vi "KickSkillVSS.vi"(8 "error in (no error)":errorcluster, 9 "BallRef":refnum<class "Ball.lvclass">, 10 "Robot":refnum<class "Robot.lvclass">, 11 "KickSkillVSS in":refnum<class "KickSkillVSS.lvclass">) -> (0 "error out":errorcluster, 2 "Robot out":refnum<class "Robot.lvclass">, 3 "KickSkillVSS out":refnum<class "KickSkillVSS.lvclass">)   [LabVIEW 2023, in "KickSkillVSS.lvclass"]
uses:
  KickSkillVSS.lvclass
  Robot_class/Robot.lvclass
  C:/Users/roboi/Downloads/VSS_AI-Larc2023/Object_class/Object.lvclass
  Ball_class/Ball.lvclass
  Field_class/Field.lvclass
  Utilities_class/Utilities.lvclass
  Object_class/Object.lvclass/Object.ctl
  Ball_class/Ball.lvclass/Ball.ctl
  Robot_class/Robot.lvclass/Robot.ctl
  Game_class/Navigation/VSSNavigation/VSSAttackerStates.ctl
  Object_class/Read x.vi
  Object_class/Read y.vi
  Ball_class/Read v_x.vi
  Ball_class/Read v_y.vi
  Object_class/Read pos_est_x.vi
  Object_class/Read pos_est_y.vi
  Robot_class/Read orientation.vi
  Robot_class/Write dest_x.vi
  Robot_class/Write dest_y.vi
  Robot_class/Write id.vi
panel:
  in  "Field":refnum<class "Field.lvclass">
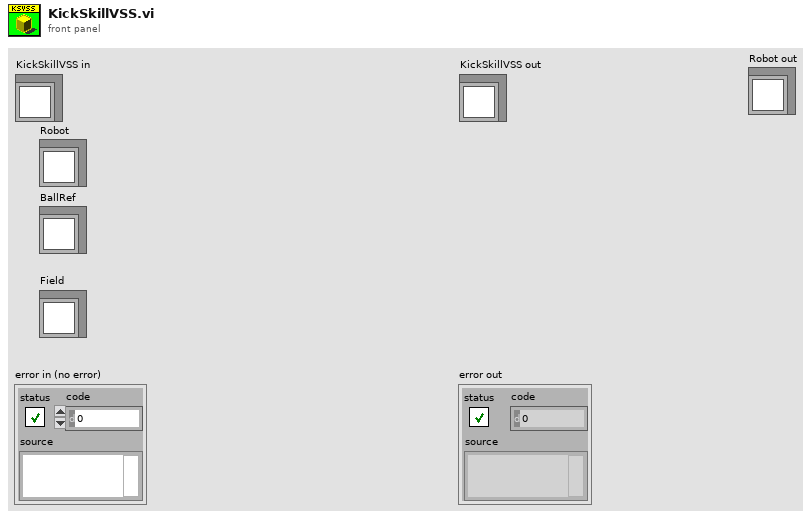
[diagram p1: front panel]
types:
  T1 = typedef "VSSAttackerStates.ctl" = enum16{"Pass", "GoToTangent", "BallGetting", "GoToKick", "Rotate anti-clockwise", "Rotate Clockwise", ""}
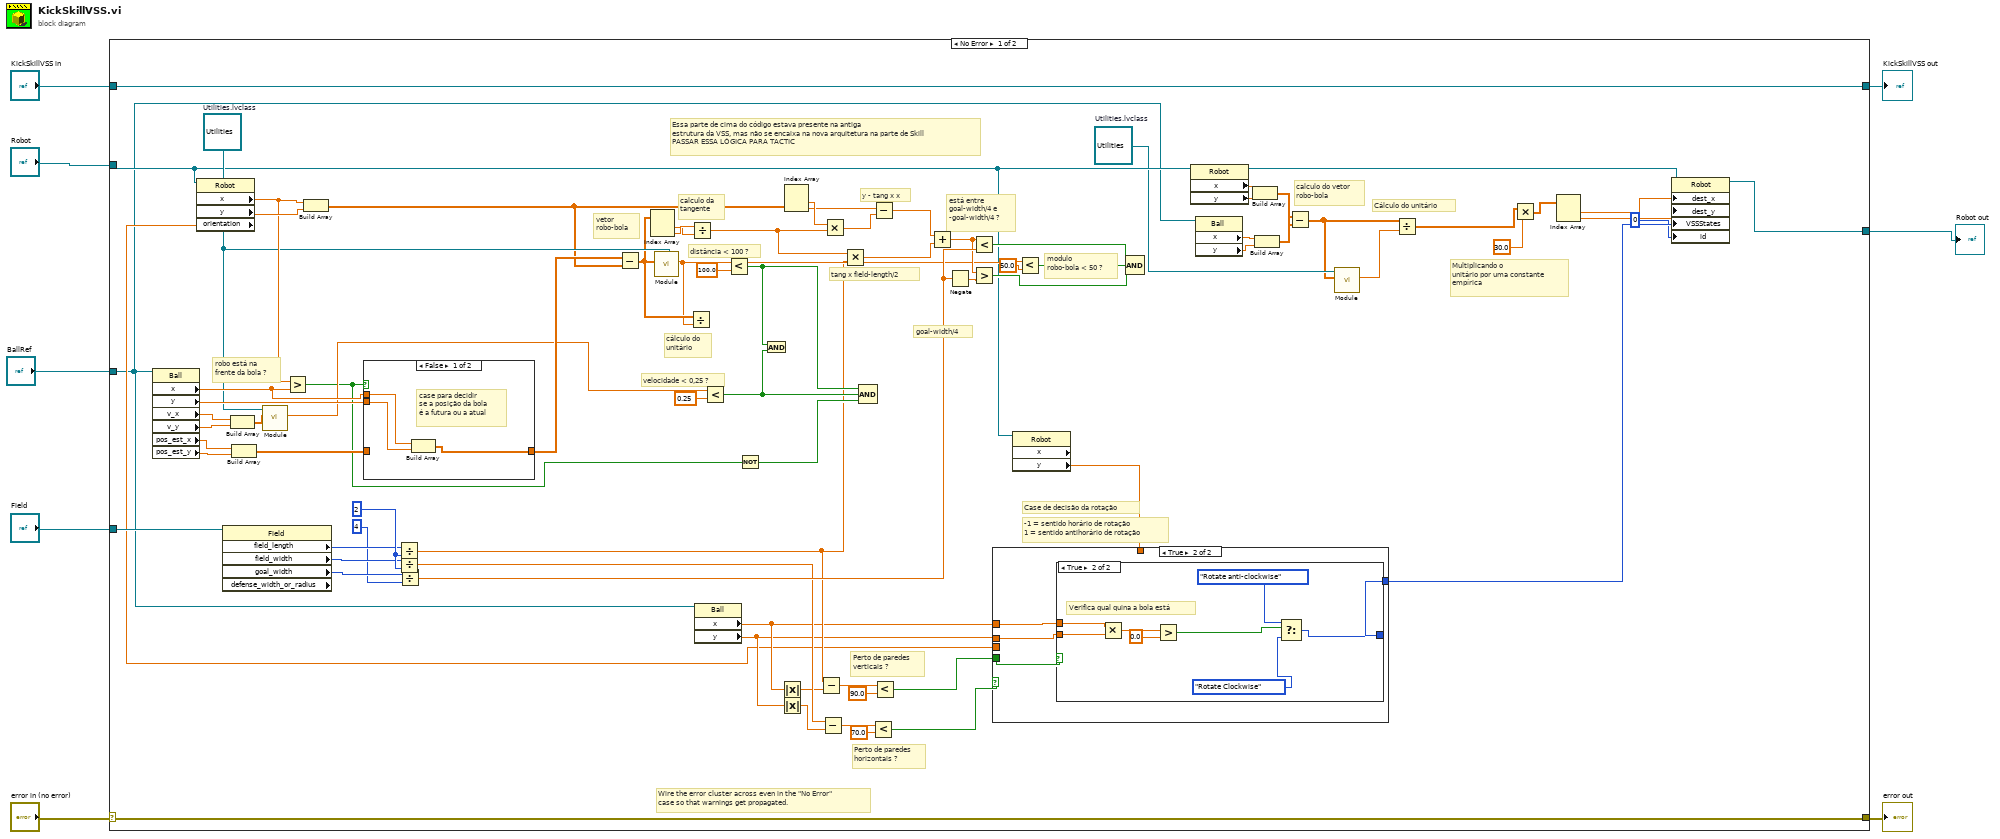
[diagram p0: block diagram]
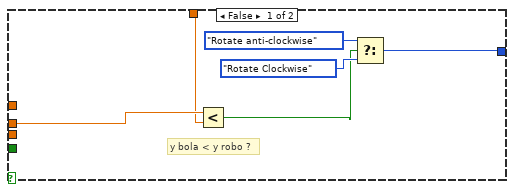
[diagram p2: hidden frame]
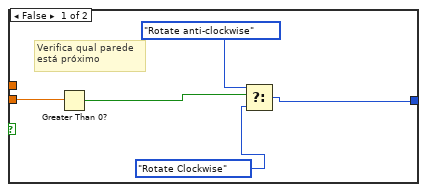
[diagram p3: hidden frame]
diagram:
  n1 = case shown="No Error" "error in (no error)" {
    selector: "error in (no error)" -> [w86 w117]
    tunnel: [w86 w117] -> w7
    tunnel: [w87 w116] -> w5
    tunnel: "KickSkillVSS in" -> [w87 w116]
    tunnel: "Robot" -> [w27 w115]
    tunnel: [w85 w115] -> w3
    tunnel: "BallRef" -> [w23 _]
    tunnel: "Field" -> [w66 _]
    frame No Error {
      w18 = refnum<class "Utilities.lvclass"> refnum  # Utilities.lvclass
      w59 = 2
      w73 = refnum<class "Utilities.lvclass"> refnum  # Utilities.lvclass
      # "Multiplicando o\nunitário por uma constante\nempírica"
      # "Cálculo do unitário"
      # "calculo do vetor\nrobo-bola"
      # "Essa parte de cima do código estava presente na antiga \nestrutura da VSS, mas não se encaixa na nova arquitetura na parte de Skill\nPASSAR ESSA LÓGICA PARA TACTIC"
      # "-1 = sentido horário de rotação\n1 = sentido antihorário de rotação"
      # "Case de decisão da rotação"
      # "Perto de paredes\nhorizontais ?"
      # "Perto de paredes\nverticais ?"
      # "modulo\nrobo-bola < 50 ?"
      # "está entre\ngoal-width/4 e\n-goal-width/4 ?"
      # "goal-width/4"
      # "y - tang x x"
      # "tang x field-length/2"
      # "velocidade < 0,25 ?"
      # "distância < 100 ?"
      # "cálculo do\nunitário"
      # "calculo da\ntangente"
      # "vetor \nrobo-bola"
      # "robo está na\nfrente da bola ?"
      # "Wire the error cluster across even in the \"No Error\"\ncase so that warnings get propagated."
      n2 = property class="Ball"(reference=w23) -> ("x"=w74:dbl, "y"=w75:dbl, "v_x"=w84:dbl, "v_y"=w83:dbl, "pos_est_x"=w81:dbl, "pos_est_y"=w80:dbl)  [unwired: 1 in, 2 out]
      n3 = property class="Robot"(reference=w27) -> ("x"=w78:dbl, "y"=w79:dbl, "orientation"=w28:dbl)  [unwired: 1 in, 2 out]
      n4 = property class="Field" props=["field_length", "field_width", "goal_width", "defense_width_or_radius"](reference=w66) -> ("field_length"=w58:i32, "field_width"=w57:i32, "goal_width"=w51:i32)  [unwired: 1 in, 3 out]
      n5 = Build Array(w84, w83) -> (w82:dbl[])
      n6 = Build Array(w81, w80) -> (w76:dbl[])
      n7 = call-dynamic "Module.vi"("2D vector"=w82, "Utilities in"=w73) -> ("Modulo"=w67:dbl)  [unwired: 7 in, 2 out]
      n8 = Greater?(x=w78, y=w74) -> (0:w64:bool)
      n9 = Build Array(w78, w79) -> (w65:dbl[])
      n10 = case shown="False" w64 {
        tunnel: [w111 w114] -> w77
        tunnel: w76 -> [_ w114]
        tunnel: w75 -> [w113 _]
        tunnel: w74 -> [w112 _]
        frame False {
          # "case para decidir \nse a posição da bola \né a futura ou a atual"
          n11 = Build Array(w112, w113) -> (w111:dbl[])
        }
        frame True {
        }
      }
      n12 = Divide(x=w58, y=w59) -> (x/y=w39:dbl)
      n13 = Divide(x=w57, y=w59) -> (x/y=w41:dbl)
      n14 = Divide(x=w51, y=4) -> (x/y=w49:dbl)
      n15 = Subtract(x=w77, y=w65) -> (x-y=w70:dbl[])
      n16 = Index Array(array=w70) -> (element #1=w71:dbl, element #2=w72:dbl)  [unwired: 2 in]
      n17 = call-dynamic "Module.vi"("2D vector"=w70, "Utilities in"=w73) -> ("Modulo"=w45:dbl)  [unwired: 7 in, 2 out]
      n18 = Divide(x=w70, y=w45) -> ()  [unwired: 1 out]
      n19 = Divide(x=w72, y=w71) -> (x/y=w60:dbl)
      n20 = property class="Ball"(reference=w23) -> ("x"=w31:dbl, "y"=w30:dbl)  [unwired: 1 in, 2 out]
      n21 = Less?(x=w67, y=0.25) -> (x < y?=w62:bool)
      n22 = Less?(x=w45, y=100.0) -> (x < y?=w63:bool)
      n23 = Not(x=w64) -> (.not. x?=w61:bool)
      n24 = And(x=w63, y=w62) -> ()  [unwired: 1 out]
      n25 = Absolute Value(x=w31) -> (abs(x)=w38:dbl)
      n26 = Absolute Value(x=w30) -> (abs(x)=w40:dbl)
      n27 = Index Array(array=w65) -> (element #1=w56:dbl, element #2=w55:dbl)  [unwired: 2 in]
      n28 = Subtract(x=w39, y=w38) -> (x-y=w37:dbl)
      n29 = Subtract(x=w41, y=w40) -> (x-y=w36:dbl)
      n30 = Multiply(x=w56, y=w60) -> (x*y=w54:dbl)
      n31 = Multiply(x=w60, y=w39) -> (x*y=w52:dbl)
      n32 = Compound Arithmetic op=AND(w63, w62, w61) -> ()  [unwired: 1 out]
      n33 = Less?(x=w36, y=70.0) -> (x < y?=w33:bool)
      n34 = Subtract(x=w55, y=w54) -> (x-y=w53:dbl)
      n35 = Less?(x=w37, y=90.0) -> (x < y?=w32:bool)
      n36 = Add(x=w53, y=w52) -> (x+y=w47:dbl)
      n37 = Negate(x=w49) -> (-x=w48:dbl)
      n38 = Less?(x=w47, y=w49) -> (x < y?=w43:bool)
      n39 = Greater?(x=w47, y=w48) -> (0:w42:bool)
      n40 = property class="Robot" props=["x", "y"](reference=w27) -> ("y"=w29:dbl)  [unwired: 1 in, 3 out]
      n41 = case shown="True" w33 {
        tunnel: w32 -> [_ w97]
        tunnel: w31 -> [_ w96]
        tunnel: w30 -> [w93 w95]
        tunnel: [w92 w94] -> w10
        tunnel: w29 -> [w91 _]
        tunnel: w28 -> [_ _]
        frame False {
          # "y bola < y robo ?"
          n42 = Less?(x=w93, y=w91) -> (x < y?=w88:bool)
          n43 = Select(t=VSSAttackerStates."Rotate anti-clockwise" ("VSSStates"), s=w88, f=VSSAttackerStates."Rotate Clockwise" ("VSSStates")) -> (s? t:f=w92:T1)
        }
        frame True {
          n44 = case shown="True" w97 {
            tunnel: w96 -> [_ w110]
            tunnel: w95 -> [w102 w109]
            tunnel: [w99 w103] -> w94
            frame False {
              # "Verifica qual parede \nestá próximo"
              n45 = Greater Than 0?(x=w102) -> (x > 0?=w100:bool)
              n46 = Select(t=VSSAttackerStates."Rotate anti-clockwise" ("VSSStates"), s=w100, f=VSSAttackerStates."Rotate Clockwise" ("VSSStates")) -> (s? t:f=w99:T1)
            }
            frame True {
              # "Verifica qual quina a bola está"
              n47 = Multiply(x=w110, y=w109) -> (x*y=w107:dbl)
              n48 = Greater?(x=w107, y=0.0) -> (0:w104:bool)
              n49 = Select(t=VSSAttackerStates."Rotate anti-clockwise" ("VSSStates"), s=w104, f=VSSAttackerStates."Rotate Clockwise" ("VSSStates")) -> (s? t:f=w103:T1)
            }
          }
        }
      }
      n50 = Less?(x=w45, y=50.0) -> (x < y?=w44:bool)
      n51 = Compound Arithmetic op=AND(w43, w44, w42) -> ()  [unwired: 1 out]
      n52 = property class="Robot"(reference=w27) -> (reference out=w26:refnum<class "Robot.lvclass">, "x"=w25:dbl, "y"=w24:dbl)  [unwired: 1 in, 1 out]
      n53 = property class="Ball"(reference=w23) -> ("x"=w22:dbl, "y"=w21:dbl)  [unwired: 1 in, 2 out]
      n54 = Build Array(w25, w24) -> (w20:dbl[])
      n55 = Build Array(w22, w21) -> (w19:dbl[])
      n56 = Subtract(x=w19, y=w20) -> (x-y=w16:dbl[])
      n57 = call-dynamic "Module.vi"("2D vector"=w16, "Utilities in"=w18) -> ("Modulo"=w17:dbl)  [unwired: 7 in, 2 out]
      n58 = Divide(x=w16, y=w17) -> (x/y=w15:dbl[])
      n59 = Multiply(x=w15, y=30.0) -> (x*y=w13:dbl[])
      n60 = Index Array(array=w13) -> (element #1=w12:dbl, element #2=w11:dbl)  [unwired: 2 in]
      n61 = property class="Robot"(reference=w26, "dest_x"=w12, "dest_y"=w11, "VSSStates"=w10, "id"=0) -> (reference out=w85:refnum<class "Robot.lvclass">)  [unwired: 1 in, 1 out]
    }
    frame Error {
    }
  }
  "error out" <- w7
  "KickSkillVSS out" <- w5
  "Robot out" <- w3
